vi "Configure TV Trigger.vi"(0 "VISA resource name":refnum<visa-resource-name>, 1 "Slope (0: Rising)":u16(ring) items=["Rising", "Falling"], 2 "Trigger Source (0: Channel 1)":u16(ring) items=["Channel 1", "Channel 2", "Channel 3", "Channel 4", "EX", "EX10"], 5 "Field Count (1)":i16=1, 7 "Field (1)":i16=1, 9 "Characteristic (0: NTSC)":u16(ring) items=["NTSC", "PALSEC", "CUST50", "CUST60"], 11 "error in (no error)":errorcluster, 12 "Number of Lines (525)":i16=525, 13 "Interlacing (2)":i16=2, 14 "Line (0)":i16) -> (4 "VISA resource name out":refnum<visa-resource-name>, 15 "error out":errorcluster)   [LabVIEW 2013, in "LeCroy Wave Series.lvlib"]
doc: "The WaveSurfer's TV triggers provide stable triggering on standard or custom composite video signals. Use them on PAL, SECAM, or NTSC systems. A composite video signal on the trigger input is analyzed to provide a signal for the beginning of the chosen field — “any,” “odd,” or “even” — and for a signal at the beginning of each line. The field signal provides the starting transition, and the beginnings of line pulses are counted to allow the final trigger on the chosen line. For each field, the number of fields, the field rate, interlace factor, and number of lines per picture must be specified — although there are standard settings for the most common types of TV signals. TV Trigger can also function in a simple any-line mode.\n\n Note:\nTV triggering in only supported for the WaveSurfer series."
uses:
  LeCroy Wave Series.lvlib
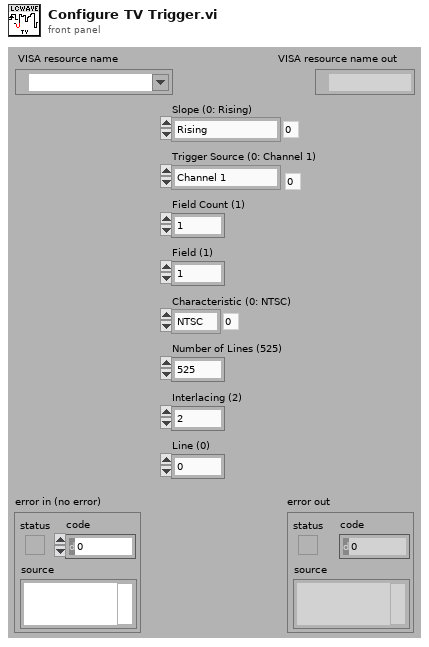
[diagram p1: front panel]
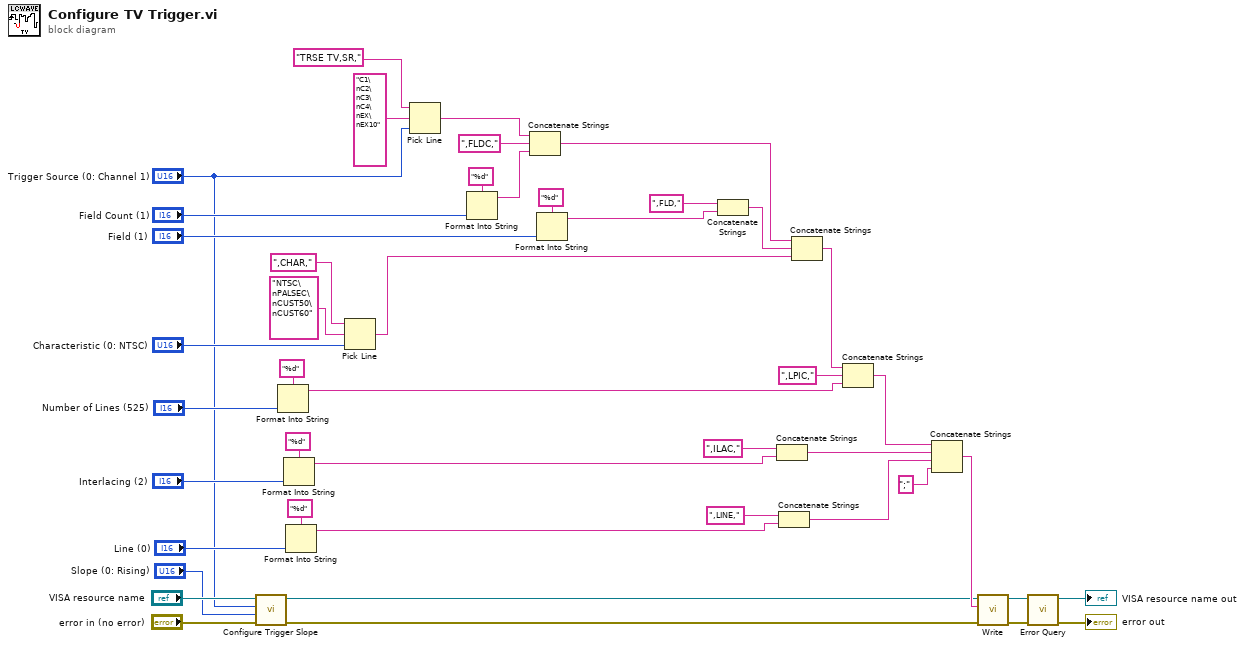
[diagram p0: block diagram]
diagram:
  n1 = call "Configure Trigger Slope.vi"("error in (no error)"="error in (no error)", "Trigger Slope (0: Rising)"="Slope (0: Rising)", "Channel (0: Channel 1)"="Trigger Source (0: Channel 1)", "VISA resource name"="VISA resource name") -> ("error out"=w3:errorcluster, "VISA resource name out"=w5:refnum<visa-resource-name>)  [unwired: 6 in]
  n2 = Format Into String(format string="%d", "Number of Lines (525)") -> (resulting string=w24:string)  [unwired: 2 in, 1 out]
  n3 = Format Into String(format string="%d", "Interlacing (2)") -> (resulting string=w19:string)  [unwired: 2 in, 1 out]
  n4 = Format Into String(format string="%d", "Line (0)") -> (resulting string=w13:string)  [unwired: 2 in, 1 out]
  n5 = Pick Line(string ("")=",CHAR,", multi-line string="NTSC\nPALSEC\nCUST50\nCUST60", line index="Characteristic (0: NTSC)") -> (output string=w28:string)
  n6 = Pick Line(string ("")="TRSE TV,SR,", multi-line string="C1\nC2\nC3\nC4\nEX\nEX10", line index="Trigger Source (0: Channel 1)") -> (output string=w36:string)
  n7 = Format Into String(format string="%d", "Field Count (1)") -> (resulting string=w37:string)  [unwired: 2 in, 1 out]
  n8 = Concatenate Strings(w36, ",FLDC," ("string"), w37) -> (w26:string)
  n9 = Format Into String(format string="%d", "Field (1)") -> (resulting string=w34:string)  [unwired: 2 in, 1 out]
  n10 = Concatenate Strings(",FLD," ("string"), w34) -> (w27:string)
  n11 = Concatenate Strings(",ILAC," ("string"), w19) -> (w16:string)
  n12 = Concatenate Strings(",LINE," ("string"), w13) -> (w10:string)
  n13 = Concatenate Strings(w26, w27, w28) -> (w21:string)
  n14 = Concatenate Strings(w21, ",LPIC," ("string"), w24) -> (w15:string)
  n15 = Concatenate Strings(w15, w16, w10, ";" ("string")) -> (w8:string)
  n16 = call "Write.vi"("error in (no error)"=w3, "Write Buffer"=w8, "VISA resource name"=w5) -> ("error out"=w42:errorcluster, "VISA resource name out"=w43:refnum<visa-resource-name>)  [unwired: 6 in, 1 out]
  n17 = call "Error Query.vi"("error in (no error)"=w42, "VISA resource name"=w43) -> ("error out"=→"error out":errorcluster, "VISA resource name out"=→"VISA resource name out":refnum<visa-resource-name>)  [unwired: 6 in, 2 out]
